vi "UpdateTestClassAfterModStopped.vi"(8 "ErrorArray In":errorcluster[](array[cluster]), 10 "Module Name":string, 11 "Test.lvclass":refnum<class "Test.lvclass">) -> (0 "ErrorArray Out":errorcluster[](array[cluster]), 2 "Module Name out":string, 3 "Test.lvclass":refnum<class "Test.lvclass">)   [LabVIEW 2018, in "Test.lvclass"]
doc: "Stops all modules based on the Test Class information (Clone Registration, Module ID, and Module list)."
uses:
  Test.lvclass
  Test.lvclass/Test.ctl
  Accessors/Write CloneReg.vi
  Accessors/Write ModuleIDs.vi
  Accessors/Write ModuleList.vi
  Accessors/Read CloneReg.vi
  Accessors/Read ModuleIDs.vi
  Accessors/Read ModuleList.vi
  <userlib>/NIST/ModuleAdminLib/CloneRegistration/CloneRegistration.lvclass
  <userlib>/NIST/NISTErrorLib/NISTErrorLib.lvlib
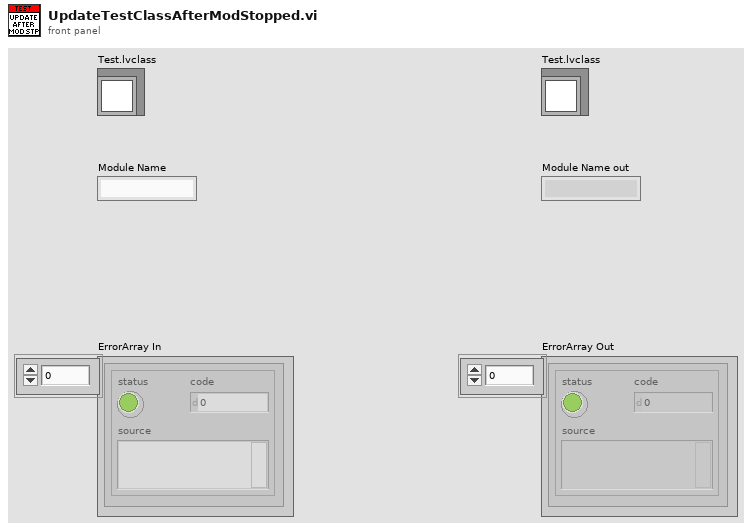
[diagram p1: front panel]
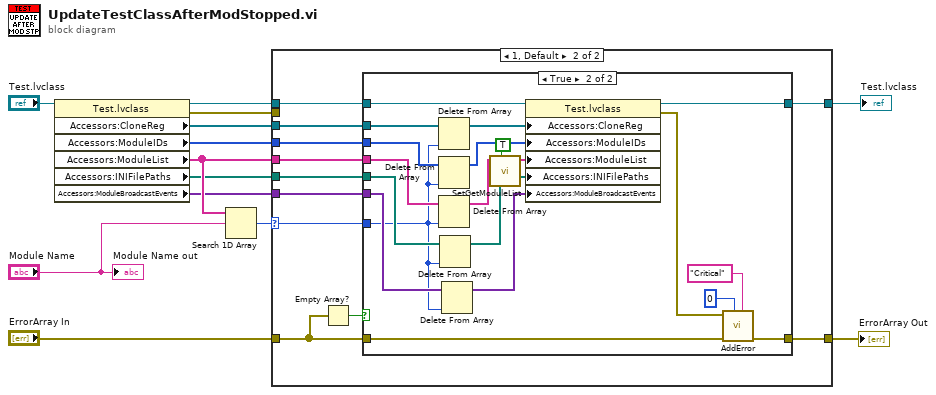
[diagram p0: block diagram]
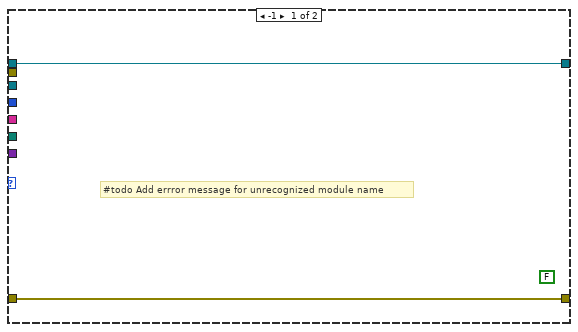
[diagram p2: hidden frame]
diagram:
  n1 = property class="Test.lvclass"(reference="Test.lvclass") -> (reference out=w9:refnum<class "Test.lvclass">, error out=w12:errorcluster, "Accessors:CloneReg"=w8:refnum<data-value>[], "Accessors:ModuleIDs"=w5:i32[], "Accessors:ModuleList"=w7:string[], "Accessors:INIFilePaths"=w2:path[], "Accessors:ModuleBroadcastEvents"=w1:variant[])  [unwired: 1 in]
  n2 = Search 1D Array(1D array=w7, element="Module Name") -> (index of element=w4:i32)  [unwired: 1 in]
  n3 = case shown="1, Default" w4 {
    selector: w4 -> [_ w20]
    tunnel: w12 -> [_ _]
    tunnel: [w14 w23] -> w11
    tunnel: "ErrorArray In" -> [w14 w16]
    tunnel: w9 -> [w15 w26]
    tunnel: w8 -> [_ w24]
    tunnel: w7 -> [_ w22]
    tunnel: w5 -> [_ w21]
    tunnel: [w15 w19] -> w3
    tunnel: w2 -> [_ w18]
    tunnel: w1 -> [_ w17]
    frame -1 {
      (unwired) FALSE ("empty?")
      # "#todo Add errror message for unrecognized module name"
    }
    frame 1, Default {
      n4 = Empty Array?(array=w16) -> (empty?=w25:bool)
      n5 = case shown="True" w25 {
        tunnel: w26 -> [w28 w48]
        tunnel: w24 -> [_ w46]
        tunnel: w21 -> [_ w45]
        tunnel: w22 -> [_ w44]
        tunnel: [w28 w47] -> w19
        tunnel: w20 -> [_ w32]
        tunnel: w16 -> [w27 w38]
        tunnel: [w27 w37] -> w23
        tunnel: w18 -> [_ w35]
        tunnel: w17 -> [_ w33]
        frame False {
        }
        frame True {
          n6 = Delete From Array(array=w46, index=w32) -> (array with subset deleted=w43:refnum<data-value>[])  [unwired: 1 in, 1 out]
          n7 = Delete From Array(array=w45, index=w32) -> (array with subset deleted=w42:i32[])  [unwired: 1 in, 1 out]
          n8 = Delete From Array(array=w44, index=w32) -> (array with subset deleted=w36:string[])  [unwired: 1 in, 1 out]
          n9 = Delete From Array(array=w35, index=w32) -> (array with subset deleted=w34:path[])  [unwired: 1 in, 1 out]
          n10 = Delete From Array(array=w33, index=w32) -> (array with subset deleted=w31:variant[])  [unwired: 1 in, 1 out]
          n11 = call "SetGetModuleList.vi"("Set? (F)"=TRUE, "ModuleList"=w36) -> ("ModuleList"=w30:string[])  [unwired: 9 in]
          n12 = property class="Test.lvclass"(reference=w48, "Accessors:CloneReg"=w43, "Accessors:ModuleIDs"=w42, "Accessors:ModuleList"=w30, "Accessors:INIFilePaths"=w34, "Accessors:ModuleBroadcastEvents"=w31) -> (reference out=w47:refnum<class "Test.lvclass">, error out=w39:errorcluster)  [unwired: 1 in]
          n13 = call <userlib>:"AddError.vi"("Severity"="Critical", "Priority"=u8 0, "ErrorArray In"=w38, "error in (no error)"=w39) -> ("ErrorArray Out"=w37:errorcluster[])  [unwired: 6 in, 1 out]
        }
      }
    }
  }
  "ErrorArray Out" <- w11
  "Test.lvclass" <- w3
  "Module Name out" <- "Module Name"
